vi "Database Transaction.vi"() -> ()   [LabVIEW 2023]
doc: "This VI demonstrates the use of transactions on a table. A transaction is begun and then a table is created in the database. The user is then prompted to decide whether or not to commit the transaction and \"write\" the changes to the database."
uses:
  <vilib>/addons/database/Auxilliary.llb/DB Tools Transaction.ctl
  <vilib>/addons/database/Auxilliary.llb/DB Tools Column Info.ctl
  <vilib>/addons/database/Auxilliary.llb/DB Tools DataTypes.ctl
  <vilib>/addons/database/Connection.llb/DB Tools Open Connec (Path).vi
  <vilib>/addons/database/Connection.llb/Conn Transaction.vi
  <vilib>/addons/database/NI_Database_API.lvlib
panel:
  out "Transaction Successful?":bool
  # "Overview: Demonstrates the use of transactions with a database.\nRequirements: Database Connectivity Toolkit\nInstructions:\n1. Run the VI.\n2. After the table is created, indicate whether or not you want to commit or rollback the transaction."
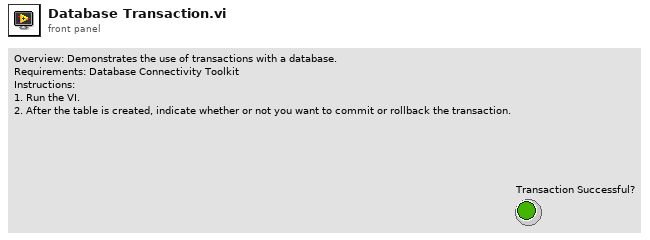
[diagram p1: front panel]
types:
  T1 = typedef "NI_Database_API.lvlib/DB Tools Column Info.ctl" = cluster{"column name":string, "data type":T2, "size":i32, "allow null?":bool}
  T2 = typedef "NI_Database_API.lvlib/DB Tools DataTypes.ctl" = enum16{"String", "Long (I32)", "Single (SGL)", "Double (DBL)", "Date/Time", "Binary"}
  T3 = typedef "NI_Database_API.lvlib/DB Tools Transaction.ctl" = enum16{"begin", "commit", "rollback"}
  T4 = typedef "NI_Database_API.lvlib/Conn ObjectReference.ctl" = refnum<k1>
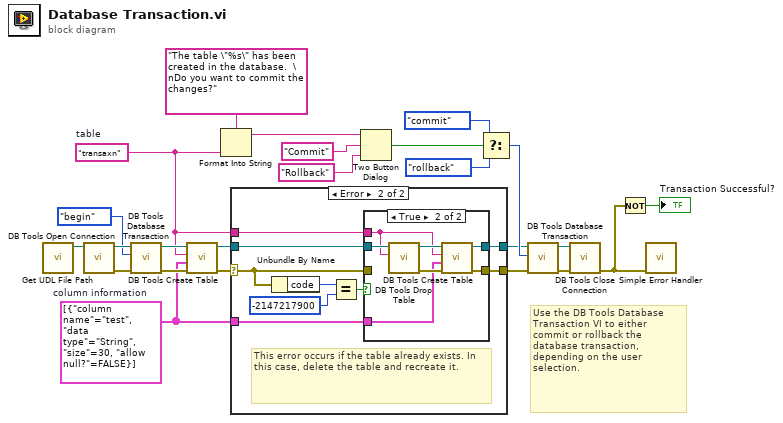
[diagram p0: block diagram]
diagram:
  w8 = T1[] [{"column name"="test", "data type"=enum."String", "size"=30, "allow null?"=FALSE}]  # column information
  w7 = "transaxn"  # table
  # "Use the DB Tools Database Transaction VI to either commit or rollback the database transaction, depending on the user selection."
  n1 = call "Get UDL File Path.vi"() -> ("UDL file path"=w15:path)  [unwired: 11 in]
  n2 = call-poly <vilib>:"DB Tools Open Connection.vi"("connection information"=w15) -> ("error out"=w24:errorcluster, "connection reference"=w23:T4)  [unwired: 7 in]
  n3 = call-poly <vilib>:"DB Tools Database Transaction.vi"("error in (no error)"=w24, "operation (begin)"=DB_Tools_Transaction."begin", "connection reference"=w23) -> ("error out"=w21:errorcluster, "connection reference out"=w20:T4)  [unwired: 3 in]
  n4 = call <vilib>:"DB Tools Create Table.vi"("error in (no error)"=w21, "column information"=w8, "table"=w7, "connection reference"=w20) -> ("error out"=w12:errorcluster, "connection reference out"=w11:T4)  [unwired: 4 in]
  n5 = Format Into String(format string="The table \"%s\" has been created in the database.  \nDo you want to commit the changes?", w7) -> (resulting string=w5:string)  [unwired: 2 in, 1 out]
  n6 = case shown="Error" w12 {
    selector: w12 -> [w25 w28]
    tunnel: w11 -> [w26 w33]
    tunnel: [w26 w32] -> w10
    tunnel: [w25 w31] -> w9
    tunnel: w7 -> [_ w30]
    tunnel: w8 -> [_ w27]
    frame No Error {
    }
    frame Error {
      # "This error occurs if the table already exists. In this case, delete the table and recreate it."
      n7 = Unbundle By Name(w28) -> ("code"=w35:i32)
      n8 = Equal?(x=w35, y=-2147217900) -> (x = y?=w29:bool)
      n9 = case shown="True" w29 {
        tunnel: w33 -> [w37 w44]
        tunnel: [w37 w39] -> w32
        tunnel: [w36 w38] -> w31
        tunnel: w30 -> [_ w41]
        tunnel: w28 -> [w36 _]
        tunnel: w27 -> [_ w40]
        frame False {
        }
        frame True {
          n10 = call <vilib>:"DB Tools Drop Table.vi"("table"=w41, "connection reference"=w44) -> ("error out"=w43:errorcluster, "connection reference out"=w42:T4)  [unwired: 6 in]
          n11 = call <vilib>:"DB Tools Create Table.vi"("error in (no error)"=w43, "column information"=w40, "table"=w41, "connection reference"=w42) -> ("error out"=w38:errorcluster, "connection reference out"=w39:T4)  [unwired: 4 in]
        }
      }
    }
  }
  n12 = Two Button Dialog(message=w5, 1:"Rollback", 2:"Commit") -> (T button?=w17:bool)
  n13 = Select(t=DB_Tools_Transaction."commit" ("operation (begin)"), s=w17, f=DB_Tools_Transaction."rollback" ("operation (begin)")) -> (s? t:f=w16:T3)
  n14 = call-poly <vilib>:"DB Tools Database Transaction.vi"("error in (no error)"=w9, "operation (begin)"=w16, "connection reference"=w10) -> ("error out"=w19:errorcluster, "connection reference out"=w18:T4)  [unwired: 3 in]
  n15 = call <vilib>:"DB Tools Close Connection.vi"("error in (no error)"=w19, "connection reference"=w18) -> ("error out"=w1:errorcluster)  [unwired: 5 in]
  n16 = Not(x=w1) -> (.not. x?=→"Transaction Successful?":bool)
  n17 = call <vilib>:"Simple Error Handler.vi"("error in (no error)"=w1) -> ()  [unwired: 4 in, 5 out]
